vi "电流插值.vi"(1 "电压":dbl[](array[numeric]), 2 "原始电压":dbl[](array[numeric]), 3 "原始电流":dbl[](array[numeric])) -> (0 "插值后电流":dbl[](array[numeric]))   [LabVIEW 2020]
uses:
  <vilib>/gmath/NI_Gmath.lvlib
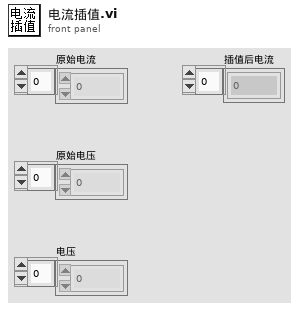
[diagram p1: front panel]
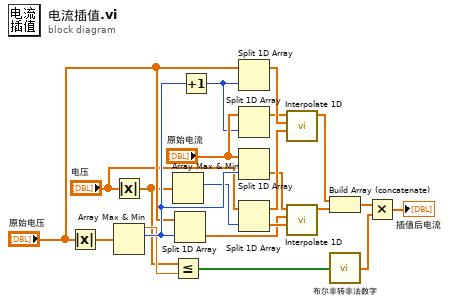
[diagram p0: block diagram]
diagram:
  n1 = Absolute Value(x="原始电压") -> (abs(x)=w2:dbl[])
  n2 = Absolute Value(x="电压") -> (abs(x)=w1:dbl[])
  n3 = Array Max & Min(array=w2) -> (max value=w10:dbl, max index (indices)=w16:i32)  [unwired: 2 out]
  n4 = Array Max & Min(array=w1) -> (max index (indices)=w5:i32)  [unwired: 3 out]
  n5 = Less Or Equal?(x=w1, y=w10) -> (x <= y?=w9:bool[])
  n6 = Split 1D Array(array="原始电压", index=w16) -> (second subarray=w18:dbl[])  [unwired: 1 out]
  n7 = Increment(x=w16) -> (x+1=w13:i32)
  n8 = Split 1D Array(array="原始电压", index=w13) -> (first subarray=w4:dbl[])  [unwired: 1 out]
  n9 = Split 1D Array(array="原始电流", index=w13) -> (first subarray=w3:dbl[])  [unwired: 1 out]
  n10 = Split 1D Array(array="原始电流", index=w16) -> (second subarray=w17:dbl[])  [unwired: 1 out]
  n11 = Split 1D Array(array="电压", index=w5) -> (first subarray=w19:dbl[], second subarray=w20:dbl[])
  n12 = call <vilib>:"Interpolate 1D.vi"("xi"=w19, "X"=w4, "Y"=w3) -> ("yi"=w6:dbl[])  [unwired: 6 in, 2 out]
  n13 = call <vilib>:"Interpolate 1D.vi"("xi"=w20, "X"=w18, "Y"=w17) -> ("yi"=w7:dbl[])  [unwired: 6 in, 2 out]
  n14 = Build Array (concatenate)(w6, w7) -> (w11:dbl[])
  n15 = call "布尔非转非法数字.vi"("布尔数组"=w9) -> ("NaN"=w8:dbl[])
  n16 = Multiply(x=w11, y=w8) -> (x*y=→"插值后电流":dbl[])
